vi "Get Frame Name.vi"(10 "Box ID":u8, 11 "Frame Name":string) -> (3 "Frame Name out":string)   [LabVIEW 2021, in "BS120x Driver.lvlib" / "BS120x.lvclass"]
uses:
  BS120x.lvclass
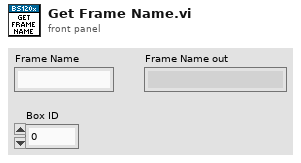
[diagram p1: front panel]
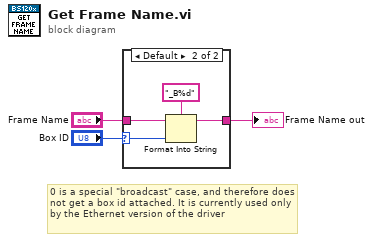
[diagram p0: block diagram]
diagram:
  # "0 is a special \"broadcast\" case, and therefore does not get a box id attached. It is currently used only by the Ethernet version of the driver"
  n1 = case shown="Default" "Box ID" {
    selector: "Box ID" -> [_ w8]
    tunnel: [w4 w7] -> w2
    tunnel: "Frame Name" -> [w4 w5]
    frame 0 {
    }
    frame Default {
      n2 = Format Into String(format string="_B%d", initial string=w5, w8) -> (resulting string=w7:string)  [unwired: 1 in, 1 out]
    }
  }
  "Frame Name out" <- w2
